vi "PicoScope4000AdvancedTriggerSettings.vi"(0 "handle in":i16, 5 "error in":errorcluster, 6 "Trigger Conditions":T4 {"Aux" items=["Don't Care", "True", "False"]; "Pulse Width Qualifier" items=["Don't Care", "True", "False"]; "Ext" items=["Don't Care", "True", "False"]; "Channel D" items=["Don't Care", "True", "False"]; "Channel C" items=["Don't Care", "True", "False"]; "Channel B" items=["Don't Care", "True", "False"]; "Channel A" items=["Don't Care", "True", "False"]; "Condition Logic" items=["AND", "OR", "XOR"]}, 8 "Channel Trigger Properties":T2 {"Channel D Trigger Properties"."Direction" items=["Above / Inside", "Below / Outside", "Rising / Enter", "Falling / Exit", "Rising or Falling / Enter or Exit", "Above Lower", "Below Lower", "Rising Lower", "Falling Lower", "Positive Runt", "Negative Runt"]; "Channel D Trigger Properties"."Threshold Mode" items=["Level", "Window"]; "Channel C Trigger Properties"."Direction" items=["Above / Inside", "Below / Outside", "Rising / Enter", "Falling / Exit", "Rising or Falling / Enter or Exit", "Above Lower", "Below Lower", "Rising Lower", "Falling Lower", "Positive Runt", "Negative Runt"]; "Channel C Trigger Properties"."Threshold Mode" items=["Level", "Window"]; "Channel B Trigger Properties"."Direction" items=["Above / Inside", "Below / Outside", "Rising / Enter", "Falling / Exit", "Rising or Falling / Enter or Exit", "Above Lower", "Below Lower", "Rising Lower", "Falling Lower", "Positive Runt", "Negative Runt"]; "Channel B Trigger Properties"."Threshold Mode" items=["Level", "Window"]; "Channel A Trigger Properties"."Direction" items=["Above / Inside", "Below / Outside", "Rising / Enter", "Falling / Exit", "Rising or Falling / Enter or Exit", "Above Lower", "Below Lower", "Rising Lower", "Falling Lower", "Positive Runt", "Negative Runt"]; "Channel A Trigger Properties"."Threshold Mode" items=["Level", "Window"]}, 9 "Addition Trigger Properties":T3 {"Aux. Trigger Properties (DO NOT USE)"."Direction" items=["Above / Inside", "Below / Outside", "Rising / Enter", "Falling / Exit", "Rising or Falling / Enter or Exit", "Above Lower", "Below Lower", "Rising Lower", "Falling Lower", "Positive Runt", "Negative Runt"]; "Aux. Trigger Properties (DO NOT USE)"."Threshold Mode" items=["Level", "Window"]; "Ext. Trigger Properties"."Direction" items=["Above / Inside", "Below / Outside", "Rising / Enter", "Falling / Exit", "Rising or Falling / Enter or Exit", "Above Lower", "Below Lower", "Rising Lower", "Falling Lower", "Positive Runt", "Negative Runt"]; "Ext. Trigger Properties"."Threshold Mode" items=["Level", "Window"]}, 10 "Auto Trigger (ms)":i32, 11 "Pulse Width Qualifier Conditions":T1 {"Aux" items=["Don't Care", "True", "False"]; "Ext" items=["Don't Care", "True", "False"]; "Channel D" items=["Don't Care", "True", "False"]; "Channel C" items=["Don't Care", "True", "False"]; "Channel B" items=["Don't Care", "True", "False"]; "Channel A" items=["Don't Care", "True", "False"]; "Condition Logic" items=["AND", "OR", "XOR"]}, 12 "Trigger Delay":u32, 13 "Pulse Width Qualifier Settings":T5 {"Pulse Width Type" items=["None", "Less Than", "Greater Than", "In Range", "Out of Range"]; "Direction" items=["Rising", "Falling", "Rising Lower", "Above", "Below", "Rising or Falling", "Falling Lower", "Below Lower", "Above Lower"]}) -> (14 "handle out":i16, 19 "error out":errorcluster)   [LabVIEW 2009]
doc: "This VI is an interface for the advanced trigger features of the oscilloscope.\nA simple trigger can be set using PicoScopeXXXXSettings.vi, in which case it is not necessary to use this VI."
uses:
  ps4000.dll
panel:
  # "For Condition Logic Suggested settings;\nFor AND, XOR logic-(parallel triggers)\nUse level-type triggers (Level or Inside/outside Window Triggers)\n\nFor OR logic- (single channel)\nUse edge types (e.g. rising, falling, entering window)"
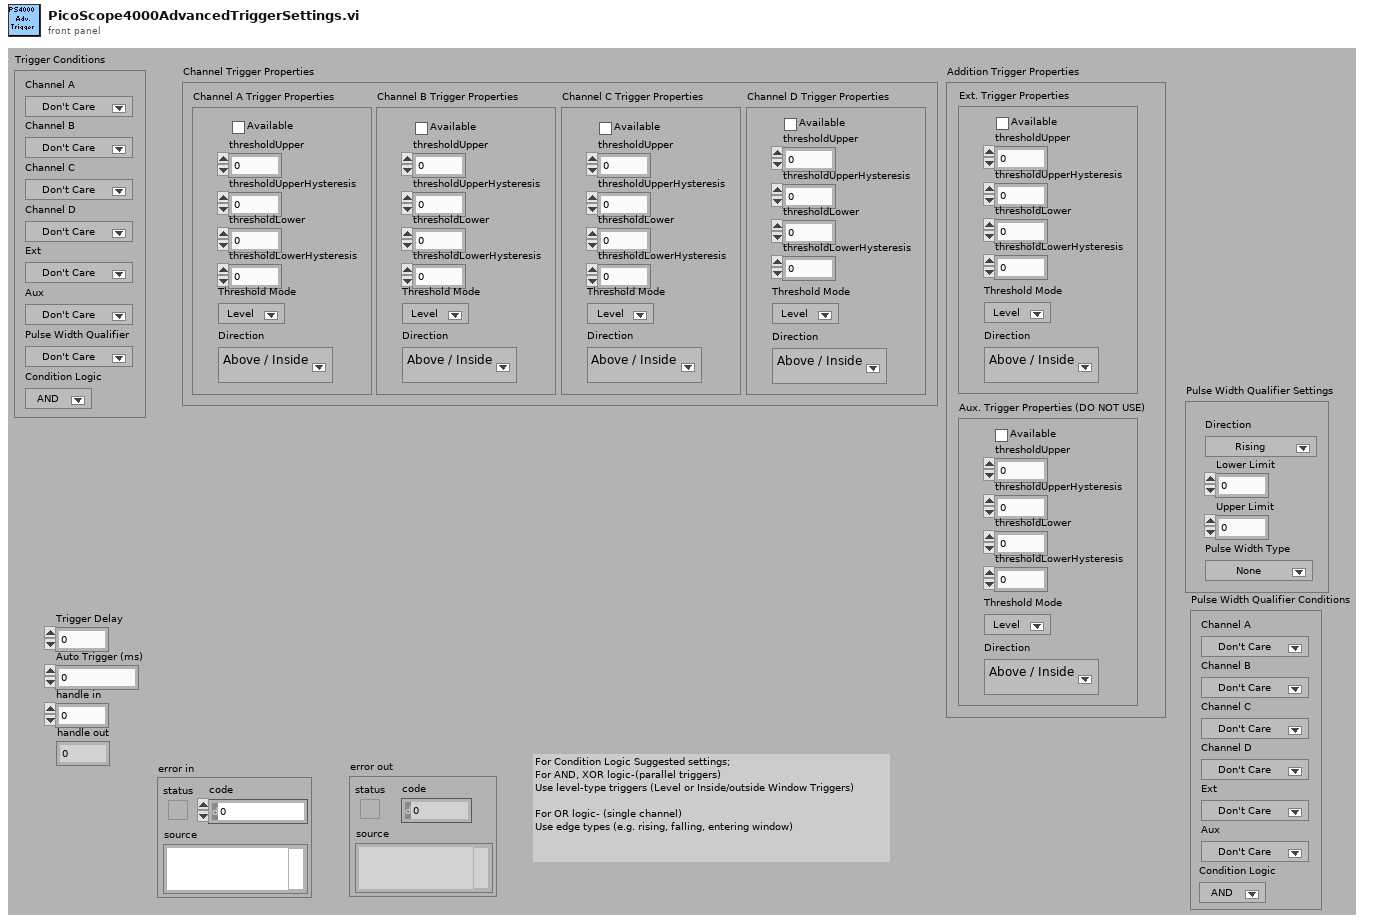
[diagram p1: front panel]
types:
  T1 = cluster{"Channel A":u16, "Channel B":u16, "Channel C":u16, "Channel D":u16, "Ext":u16, "Aux":u16, "Condition Logic":u16}
  T2 = cluster{"Channel A Trigger Properties":cluster{"thresholdUpper":i16, "thresholdUpperHysteresis":u16, "thresholdLower":i16, "thresholdLowerHysteresis":u16, "Threshold Mode":i32, "Direction":u32, "Available":bool}, "Channel B Trigger Properties":cluster{"thresholdUpper":i16, "thresholdUpperHysteresis":u16, "thresholdLower":i16, "thresholdLowerHysteresis":u16, "Threshold Mode":i32, "Direction":u32, "Available":bool}, "Channel C Trigger Properties":cluster{"thresholdUpper":i16, "thresholdUpperHysteresis":u16, "thresholdLower":i16, "thresholdLowerHysteresis":u16, "Threshold Mode":i32, "Direction":u32, "Available":bool}, "Channel D Trigger Properties":cluster{"thresholdUpper":i16, "thresholdUpperHysteresis":u16, "thresholdLower":i16, "thresholdLowerHysteresis":u16, "Threshold Mode":i32, "Direction":u32, "Available":bool}}
  T3 = cluster{"Ext. Trigger Properties":cluster{"thresholdUpper":i16, "thresholdUpperHysteresis":u16, "thresholdLower":i16, "thresholdLowerHysteresis":u16, "Threshold Mode":i32, "Direction":u32, "Available":bool}, "Aux. Trigger Properties (DO NOT USE)":cluster{"thresholdUpper":i16, "thresholdUpperHysteresis":u16, "thresholdLower":i16, "thresholdLowerHysteresis":u16, "Threshold Mode":i32, "Direction":u32, "Available":bool}}
  T4 = cluster{"Channel A":u16, "Channel B":u16, "Channel C":u16, "Channel D":u16, "Ext":u16, "Aux":u16, "Pulse Width Qualifier":u16, "Condition Logic":u16}
  T5 = cluster{"Direction":u32, "Lower Limit":u32, "Upper Limit":u32, "Pulse Width Type":u32}
  T6 = cluster{"thresholdUpper":i16, "thresholdUpperHysteresis":u16, "thresholdLower":i16, "thresholdLowerHysteresis":u16, "Threshold Mode":i32, "Direction":u32, "Available":bool}[]
  T7 = cluster{"[0]":u32, "[1]":u32, "[2]":u32, "[3]":u32, "[4]":u32, "[5]":u32, "[6]":u32, "[7]":u32, "[8]":u32}
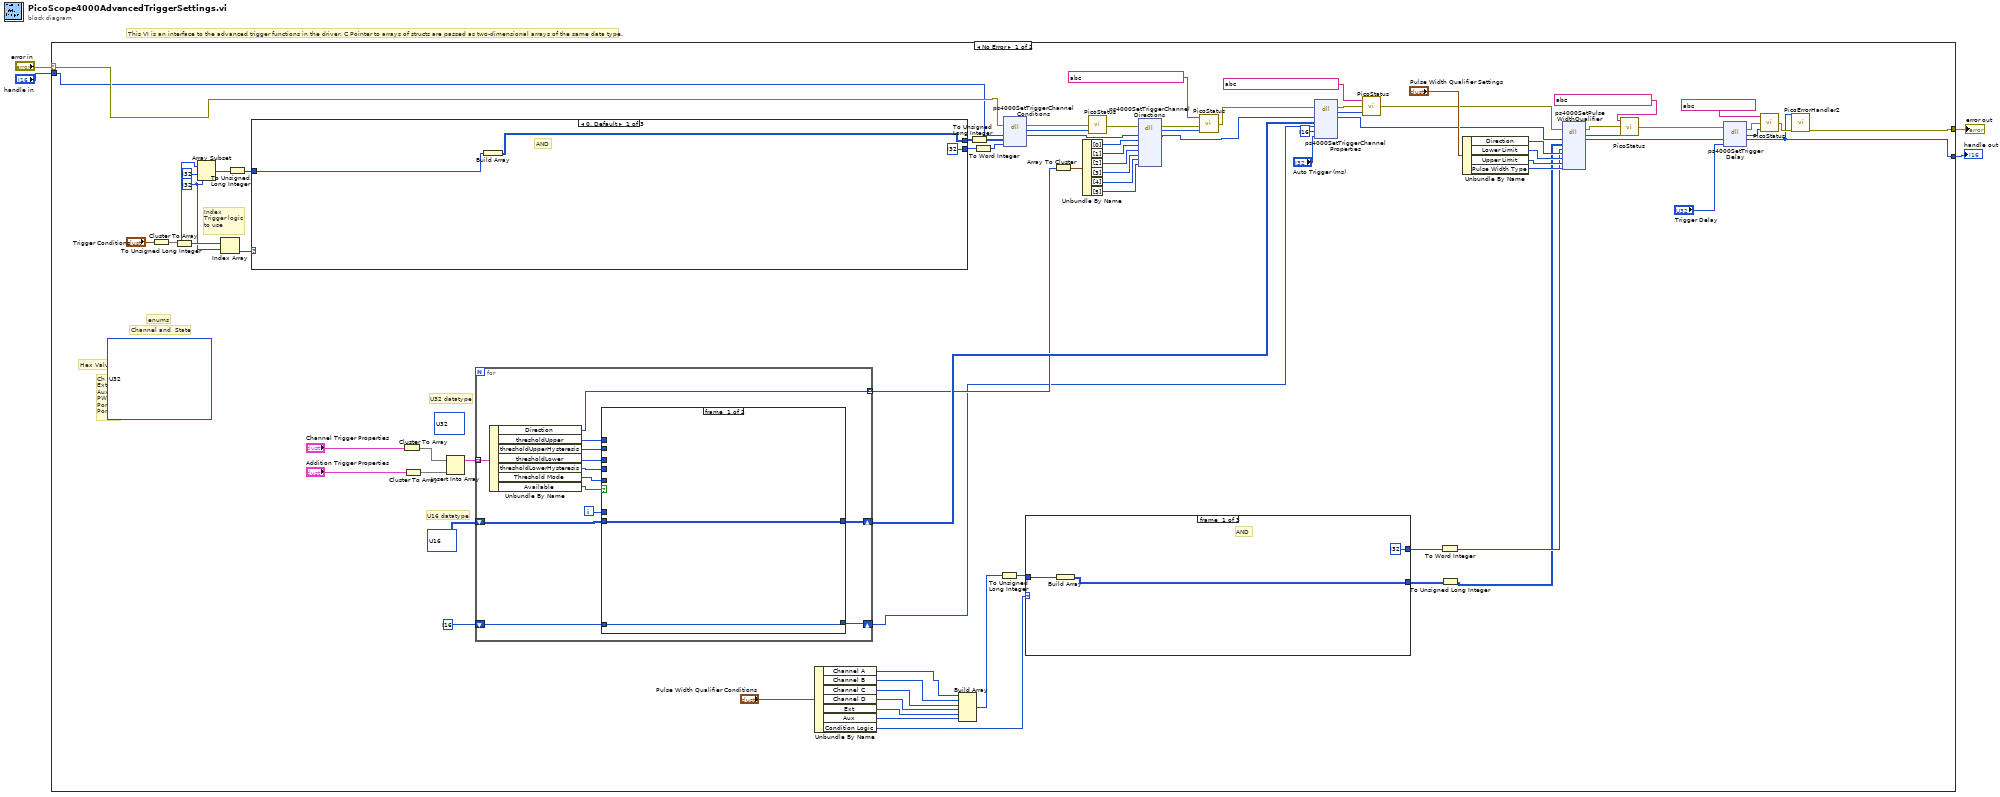
[diagram p0: block diagram]
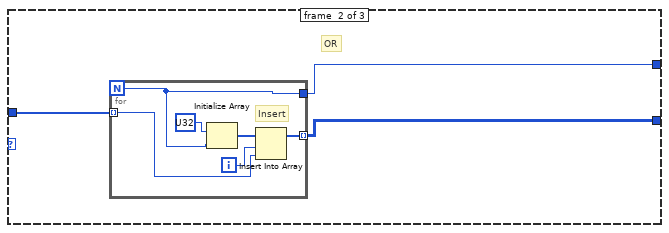
[diagram p2: hidden frame]
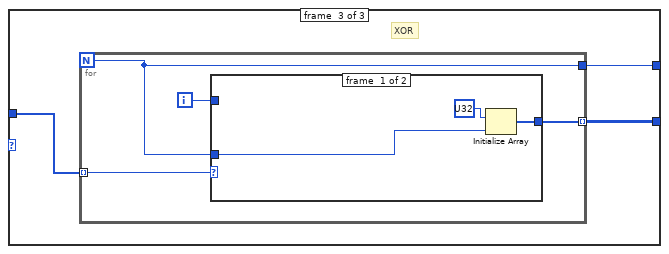
[diagram p3: hidden frame]
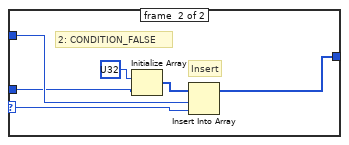
[diagram p4: hidden frame]
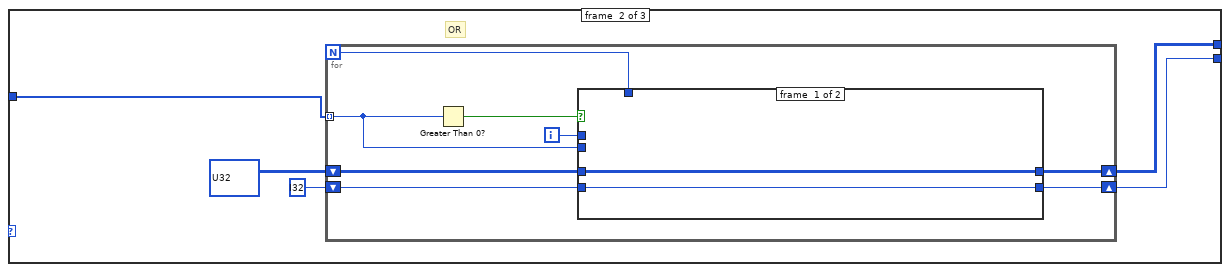
[diagram p5: hidden frame]
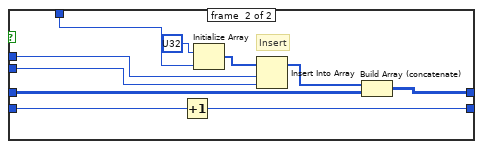
[diagram p6: hidden frame]
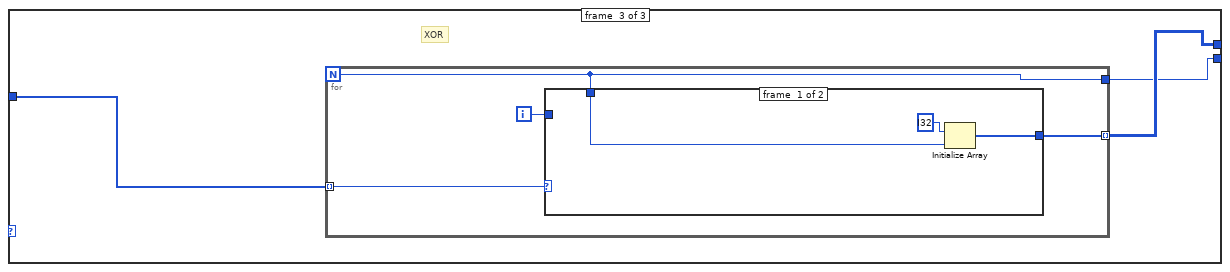
[diagram p7: hidden frame]
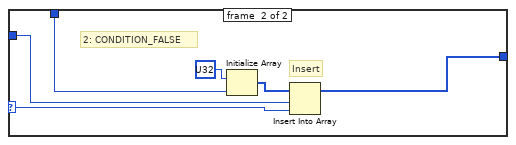
[diagram p8: hidden frame]
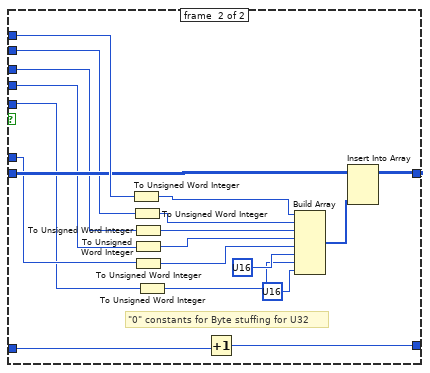
[diagram p9: hidden frame]
diagram:
  # "This VI is an interface to the advanced trigger functions in the driver. C Pointer to arrays of structs are passed as two-dimensional arrays of the same data type."
  n1 = case shown="No Error" "error in" {
    selector: "error in" -> [w30 w189]
    tunnel: "handle in" -> [w29 w190]
    tunnel: [w71 w190] -> w2
    tunnel: [w72 w189] -> w1
    frame #0 {
      w5 = i32 ? ("length")
      (unwired) u32[][] ?
      (unwired) u32[][] ?
      # "Index\nTrigger logic\nto use"
      # "enums"
      # "Ch D\nExt\nAux\nPWQ\nPort0\nPort1"
      # "Channel and  State"
      # "Hex Values"
      # "U16 datatype"
      # "U32 datatype"
      n2 = Cluster To Array(cluster="Trigger Conditions") -> (array=w74:u16[])
      n3 = To Unsigned Long Integer(number=w74) -> (unsigned 32bit integer=w21:u32[])
      n4 = Array Subset(array=w21, index=i32 ?, length=w5) -> (w23:u32[])
      n5 = Index Array(array=w21, index=w5) -> (element=w34:u32)
      n6 = To Unsigned Long Integer(number=w23) -> (unsigned 32bit integer=w22:u32[])
      n7 = case shown="0, Default" w34 {
        tunnel: [w113 w118 w141] -> w27
        tunnel: [i32 ? w114 w139] -> w26
        tunnel: w22 -> [w112 w115 w140]
        frame #0 {
          # "AND"
          n8 = Build Array(w112) -> (w113:u32[][])
        }
        frame #1 {
          # "OR"
          n9 = for {
            N -> [w119]
            tunnel: w115 -> [w123] mode=indexing
            shift-right: [w122] -> w118
            shift-left: u32[][] ? -> [w126]
            shift-right: [w120] -> w114
            shift-left: i32 ? -> [w121]
            i -> [w125]
            n10 = Greater Than 0?(x=w123) -> (x > 0?=w124:bool)
            n11 = case shown="True" w124 {
              tunnel: w126 -> [w128 w132]
              tunnel: w125 -> [_ w136]
              tunnel: w123 -> [_ w135]
              tunnel: [w128 w134] -> w122
              tunnel: w121 -> [w127 w131]
              tunnel: [w127 w130] -> w120
              tunnel: w119 -> [_ w129]
              frame #0 {
              }
              frame #1 {
                # "Insert"
                n12 = Increment(x=w131) -> (x+1=w130:i32)
                n13 = Initialize Array(u32 ? ("element"), w129) -> (w137:u32[])
                n14 = Insert Into Array(array=w137, index=w136, new element=w135) -> (w133:u32[])
                n15 = Build Array (concatenate)(w133, w132) -> (w134:u32[][])
              }
            }
          }
        }
        frame #2 {
          # "XOR"
          n16 = for {
            N -> [w142]
            tunnel: w140 -> [w143] mode=indexing
            tunnel: [w145] -> w141 mode=indexing
            tunnel: [w142] -> w139
            i -> [w144]
            n17 = case shown="1" w143 {
              selector: w143 -> [_ w151]
              tunnel: [w147 w152] -> w145
              tunnel: w144 -> [_ w150]
              tunnel: w142 -> [w146 w149]
              frame #0 {
                n18 = Initialize Array(i32 ? ("element"), w146) -> (w147:i32[])
              }
              frame #1 {
                # "2: CONDITION_FALSE"
                # "Insert"
                n19 = Initialize Array(u32 ? ("element"), w149) -> (w153:u32[])
                n20 = Insert Into Array(array=w153, index=w150, new element=w151) -> (w152:u32[])
              }
            }
          }
        }
      }
      n21 = Cluster To Array(cluster="Channel Trigger Properties") -> (array=w66:T6)
      n22 = Cluster To Array(cluster="Addition Trigger Properties") -> (array=w64:T6)
      n23 = Insert Into Array(array=w66, new element=w64) -> (w65:T6)  [unwired: 1 in]
      n24 = for {
        tunnel: w65 -> [w158] mode=indexing
        shift-right: [w159] -> w42
        shift-left: u16[][] ? -> [w160]
        tunnel: [w157] -> w41 mode=indexing
        shift-right: [w155] -> w37
        shift-left: i16 ? -> [w156]
        i -> [w161]
        n25 = Unbundle By Name(w158) -> ("Direction"=w157:u32, "thresholdUpper"=w167:i16, "thresholdUpperHysteresis"=w166:u16, "thresholdLower"=w165:i16, "thresholdLowerHysteresis"=w164:u16, "Threshold Mode"=w163:i32, "Available"=w162:bool)
        n26 = case shown="True" w162 {
          tunnel: w167 -> [_ w188]
          tunnel: w166 -> [_ w178]
          tunnel: w165 -> [_ w177]
          tunnel: w164 -> [_ w176]
          tunnel: w163 -> [_ w172]
          tunnel: w161 -> [_ w183]
          tunnel: [w169 w185] -> w159
          tunnel: w160 -> [w169 w184]
          tunnel: w156 -> [w168 w171]
          tunnel: [w168 w170] -> w155
          frame #0 {
          }
          frame #1 {
            # "\"0\" constants for Byte stuffing for U32"
            n27 = To Unsigned Word Integer(number=w188) -> (unsigned 16bit integer=w180:u16)
            n28 = To Unsigned Word Integer(number=w178) -> (unsigned 16bit integer=w179:u16)
            n29 = To Unsigned Word Integer(number=w177) -> (unsigned 16bit integer=w175:u16)
            n30 = To Unsigned Word Integer(number=w176) -> (unsigned 16bit integer=w181:u16)
            n31 = To Unsigned Word Integer(number=w183) -> (unsigned 16bit integer=w182:u16)
            n32 = To Unsigned Word Integer(number=w172) -> (unsigned 16bit integer=w173:u16)
            n33 = Increment(x=w171) -> (x+1=w170:i16)
            n34 = Build Array(w180, w179, w175, w181, w182, u16 ? ("element"), w173, u16 ? ("element")) -> (w186:u16[])
            n35 = Insert Into Array(array=w184, new element=w186) -> (w185:u16[][])  [unwired: 2 in]
          }
        }
      }
      n36 = Unbundle By Name("Pulse Width Qualifier Conditions") -> ("Channel A"=w63:u16, "Channel B"=w62:u16, "Channel C"=w61:u16, "Channel D"=w60:u16, "Ext"=w58:u16, "Aux"=w57:u16, "Condition Logic"=w19:u16)
      n37 = Build Array(w63, w62, w61, w60, w58, w57) -> (w73:u16[])
      n38 = To Unsigned Long Integer(number=w27) -> (unsigned 32bit integer=w28:u32[][])
      n39 = To Word Integer(number=w26) -> (16bit integer=w25:i16)
      n40 = To Unsigned Long Integer(number=w73) -> (unsigned 32bit integer=w20:u32[])
      n41 = dll-call lib="ps4000.dll" fn="ps4000SetTriggerChannelConditions" ("ps3000.dll:_ps3000_open_unit@0")(error in=w30, "handle"=w29, "conditions"=w28, "nConditions"=w25) -> (error out=w33:errorcluster, "PICO_STATUS"=w32:u32, "handle"=w31:i16)  [unwired: 4 in, 1 out]
      n42 = case shown="1" w19 {
        tunnel: [w85 w88 w97] -> w18
        tunnel: [i32 ? w87 w96] -> w17
        tunnel: w20 -> [w84 w86 w95]
        frame #0 {
          # "AND"
          n43 = Build Array(w84) -> (w85:u32[][])
        }
        frame #1 {
          # "OR"
          n44 = for {
            N -> [w89]
            tunnel: w86 -> [w91] mode=indexing
            tunnel: [w90] -> w88 mode=indexing
            tunnel: [w89] -> w87
            i -> [w92]
            # "Insert"
            n45 = Initialize Array(u32 ? ("element"), w89) -> (w93:u32[])
            n46 = Insert Into Array(array=w93, index=w92, new element=w91) -> (w90:u32[])
          }
        }
        frame #2 {
          # "XOR"
          n47 = for {
            N -> [w98]
            tunnel: w95 -> [w101] mode=indexing
            tunnel: [w99] -> w97 mode=indexing
            tunnel: [w98] -> w96
            i -> [w100]
            n48 = case shown="1" w101 {
              selector: w101 -> [_ w107]
              tunnel: [w103 w108] -> w99
              tunnel: w100 -> [_ w106]
              tunnel: w98 -> [w102 w105]
              frame #0 {
                n49 = Initialize Array(u32 ? ("element"), w102) -> (w103:u32[])
              }
              frame #1 {
                # "2: CONDITION_FALSE"
                # "Insert"
                n50 = Initialize Array(u32 ? ("element"), w105) -> (w109:u32[])
                n51 = Insert Into Array(array=w109, index=w106, new element=w107) -> (w108:u32[])
              }
            }
          }
        }
      }
      n52 = Array To Cluster(array=w41) -> (cluster=w52:T7)
      n53 = Unbundle By Name(w52) -> ("[0]"=w51:u32, "[1]"=w50:u32, "[2]"=w49:u32, "[3]"=w48:u32, "[4]"=w47:u32, "[5]"=w46:u32)
      n54 = call "PicoStatus.vi"("PICO STATUS"=w32, "error in"=w33) -> ("error out"=w54:errorcluster)  [unwired: 1 in]
      n55 = dll-call lib="ps4000.dll" fn="ps4000SetTriggerChannelDirections" ("ps3000.dll:_ps3000_open_unit@0")(error in=w54, "handle"=w31, "channelA"=w51, "channelB"=w50, "channelC"=w49, "channelD"=w48, "ext"=w47, "aux"=w46) -> (error out=w55:errorcluster, "PICO_STATUS"=w53:u32, "handle"=w39:i16)  [unwired: 8 in, 1 out]
      n56 = call "PicoStatus.vi"("PICO STATUS"=w53, "error in"=w55, "source"=string ?) -> ("error out"=w40:errorcluster)
      n57 = dll-call lib="ps4000.dll" fn="ps4000SetTriggerChannelProperties" ("ps3000.dll:_ps3000_open_unit@0")(error in=w40, "handle"=w39, "channelProperties"=w42, "nChannelProperties"=w37, "auxOutputEnable"=i16 ?, "autoTriggerMilliseconds"="Auto Trigger (ms)") -> (error out=w44:errorcluster, "PICO_STATUS"=w45:u32, "handle"=w10:i16)  [unwired: 6 in, 1 out]
      n58 = call "PicoStatus.vi"("PICO STATUS"=w45, "error in"=w44, "source"=string ?) -> ("error out"=w8:errorcluster)
      n59 = To Word Integer(number=w17) -> (16bit integer=w12:i16)
      n60 = To Unsigned Long Integer(number=w18) -> (unsigned 32bit integer=w11:u32[][])
      n61 = Unbundle By Name("Pulse Width Qualifier Settings") -> ("Direction"=w16:u32, "Lower Limit"=w15:u32, "Upper Limit"=w14:u32, "Pulse Width Type"=w13:u32)
      n62 = dll-call lib="ps4000.dll" fn="ps4000SetPulseWidthQualifier" ("ps3000.dll:_ps3000_open_unit@0")(error in=w8, "handle"=w10, "conditions"=w11, "nConditions"=w12, "direction"=w16, "lower"=w15, "upper"=w14, "type"=w13) -> (error out=w9:errorcluster, "PICO_STATUS"=w7:u32, "handle"=w6:i16)  [unwired: 8 in, 1 out]
      n63 = call "PicoStatus.vi"("PICO STATUS"=w7, "error in"=w9, "source"=string ?) -> ("error out"=w69:errorcluster)
      n64 = dll-call lib="ps4000.dll" fn="ps4000SetTriggerDelay" ("ps3000.dll:_ps3000_open_unit@0")(error in=w69, "handle"=w6, "delay"="Trigger Delay") -> (error out=w80:errorcluster, "PICO_STATUS"=w81:u32, "handle"=w71:i16)  [unwired: 3 in, 1 out]
      n65 = call "PicoStatus.vi"("PICO STATUS"=w81, "error in"=w80, "source"=string ?) -> ("error out"=w79:errorcluster)
      n66 = call "PicoErrorHandler2.vi"("error in (no error)"=w79, "handle In"=w71) -> ("error out"=w72:errorcluster)  [unwired: 9 in]
    }
    frame #1 {
    }
  }
  "handle out" <- w2
  "error out" <- w1
